vi "Draw Template Glyph.vi"(10 "Rectangle dimension (32,32)":T1, 11 "Rectangle colors (black, white)":T2) -> (3 "Template Glyph":picture)   [LabVIEW 2021, in "LabVIEW Icon API.lvlib"]
doc: "Draw a rectangle based on the passed in data."
uses:
  LabVIEW Icon API.lvlib
  API_Rectangle Colors.ctl
  API_Rectangle Dimension.ctl
  lv_icon/lv_icon.lvlib
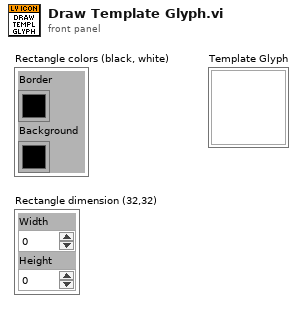
[diagram p1: front panel]
types:
  T1 = typedef "LabVIEW Icon API.lvlib/API_Rectangle Dimension.ctl" = cluster{"Width":i16, "Height":i16}
  T2 = typedef "LabVIEW Icon API.lvlib/API_Rectangle Colors.ctl" = cluster{"Border":u32, "Background":u32}
  T3 = cluster{"left":i16, "top":i16, "right":i16, "bottom":i16}
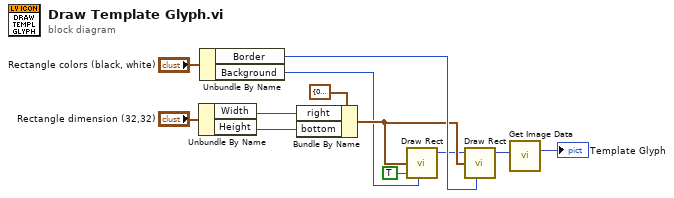
[diagram p0: block diagram]
diagram:
  n1 = Unbundle By Name("Rectangle dimension (32,32)") -> ("Width"=w3:i16, "Height"=w4:i16)
  n2 = Unbundle By Name("Rectangle colors (black, white)") -> ("Border"=w10:u32, "Background"=w7:u32)
  n3 = Bundle By Name(cluster=T3 {"left"=0, "top"=0, "right"=0, "bottom"=0} ("rect"), "right"=w3, "bottom"=w4) -> (w9:T3)
  n4 = call <vilib>:"Draw Rect.vi"("rect"=w9, "fill?(F)"=TRUE, "color(black)"=w7) -> ("new picture"=w8:picture)  [unwired: 6 in]
  n5 = call <vilib>:"Draw Rect.vi"("picture"=w8, "rect"=w9, "color(black)"=w10) -> ("new picture"=w11:picture)  [unwired: 6 in]
  n6 = call "Get Image Data.vi"("Pic In"=w11) -> ("Pic Out"=→"Template Glyph":picture)  [unwired: 2 in, 8 out]
